vi "PointDetection-AnyPath.vi"() -> ()   [LabVIEW 2014]
doc: "This example shows how to use the Edge Tool in NI Vision. The Edge Tool finds edges (or sharp transitions in the pixels values) along a given line or ROI profile. The Edge Tool is a precursor function to many of the gauging and inspection tasks. For example, the location of the edges found along a line profile across an object can interpreted as the boundaries of the object whose dimensions have to be measured for a gauging application or the presence of a crack in the surface of an object for an inspection application."
uses:
  <vilib>/vision/NI_Vision_Development_Module.lvlib
panel:
  out "Number of Edges Detected":i32
  in  "Process":u16(ring)=2 items=["Get First Edge", "Get First + Last Edge", "Get All Edges", "Get Best Edge"]
  in  "Edge Options":T1={"Edge Polarity"=0, "Kernel Size"=3, "Width"=5, "Minimum Edge Strength"=10.0, "Interpolation Type"=1, "Data Processing Method"=0} {"Data Processing Method" items=["Average", "Median"]; "Interpolation Type" items=["Zero Order"=0, "Bilinear"=1, "Bilinear Fixed"=4]; "Minimum Edge Strength" min=0.0 max=255.0 format="%.2g"; "Width" min=1 step=2; "Kernel Size" min=3 step=2; "Edge Polarity" items=["All Edges", "Rising Edges", "Falling Edges"]}
  out "Gradient Information":dbl[](graph)
  out "Image":T2(plugin-control)
  out "Line Profile":cluster{"x0":sgl, "dx":sgl, "Pixels Line":sgl[]}(graph)
  in  "Stop":bool
  # "Overview: Demonstrates the edges detection along a Region of Interest (ROI).\nRequirements: Vision Development Software.\nInstructions: 1. Run the VI;  2. Change the Process or Edge Options to see the edges detected along the ROI."
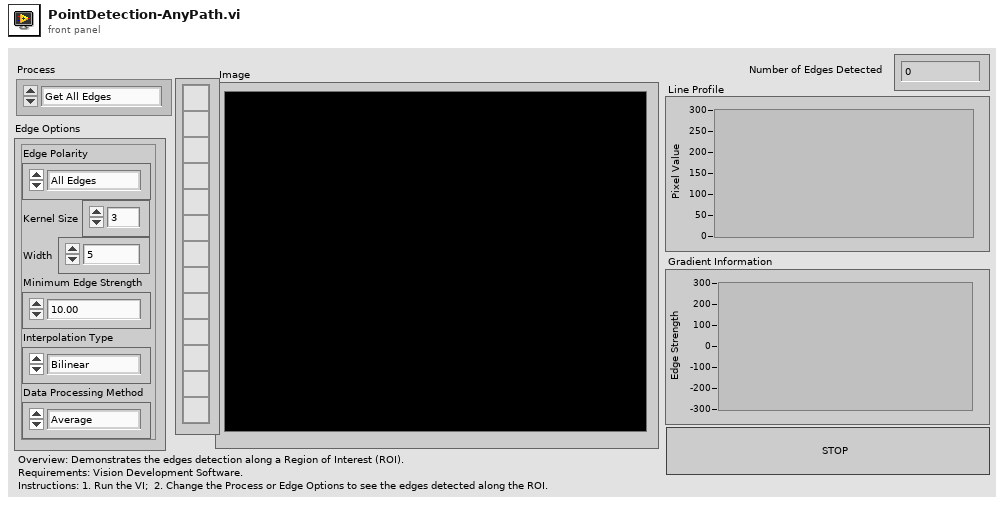
[diagram p1: front panel]
types:
  T1 = cluster{"Edge Polarity":u16, "Kernel Size":u32, "Width":u32, "Minimum Edge Strength":dbl, "Interpolation Type":u16, "Data Processing Method":u16}
  T2 = typedef "IMAQ Image.ctl" = refnum<image>
  T3 = typedef "IMAQ Line" = cluster{"Start X":i32, "Start Y":i32, "End X":i32, "End Y":i32}
  T4 = typedef "ROI Descriptor" = cluster{"Global Rectangle":i32[], "Contours":cluster{"ID":enum32{"External", "Internal"}, "Type":u32, "Coordinates":i32[]}[]}
  T5 = cluster{"Global Rectangle":i32[], "Contours":cluster{"Contour Type":u32, "ROI Type":u32, "Points":i32[]}[]}
  T6 = typedef "Edge New.ctl" = cluster{"Location (Pixel)":cluster{"X":sgl, "Y":sgl}, "Location (Real-World)":cluster{"X":sgl, "Y":sgl}, "Distance (Pixel)":dbl, "Distance (Real-World)":dbl, "Strength":dbl, "Noise":dbl, "Rising?":bool}
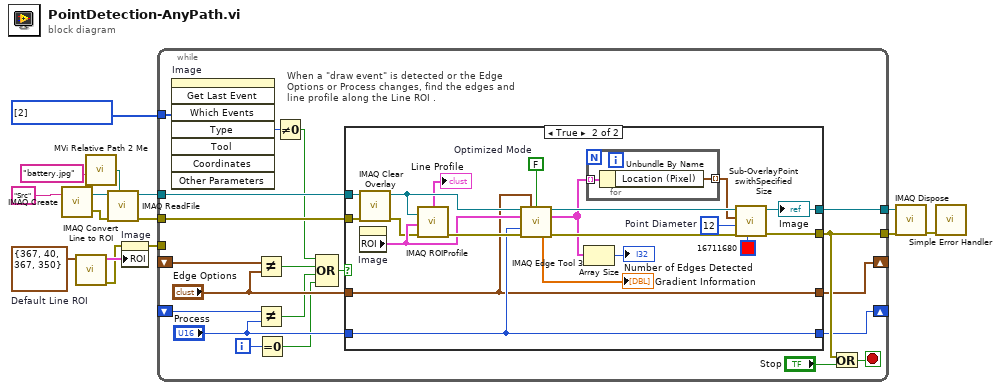
[diagram p0: block diagram]
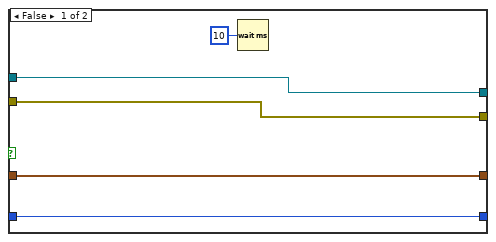
[diagram p2: hidden frame]
diagram:
  w3 = T3 {"Start X"=367, "Start Y"=40, "End X"=367, "End Y"=350}  # Default Line ROI
  w7 = i32[] [2] items=["No  event", "Click event", "Draw event", "Move event", "Size event", "Scroll event", "Activate event", "Close event", "Double click event"] ("Events list (all)")
  n1 = call "IMAQ Create"("Image Name"="Src") -> ("New Image"=w14:T2, "error out"=w13:errorcluster)  [unwired: 4 in]
  n2 = call "IMAQ Convert Line to ROI"("Line"=w3) -> ("error out"=w1:errorcluster, "ROI Descriptor"=w2:T4)  [unwired: 8 in]
  n3 = call "MVi Relative Path 2 Me.vi"("Relative Path"="battery.jpg" ("name or relative path")) -> ("Appended Dir"=w4:path)  [unwired: 5 in, 1 out]
  n4 = call "IMAQ ReadFile"("File Path"=w4, "error in (no error)"=w13, "Image"=w14) -> ("error out"=w8:errorcluster, "Image Out"=w9:T2)  [unwired: 4 in, 3 out]
  n5 = property on="Image" class="ImageControl"(error in=w1, "ROI"=w2) -> (error out=w6:errorcluster)  [unwired: 1 in, 1 out]
  n6 = while {
    tunnel: w9 -> [w34]
    tunnel: w8 -> [w35]
    tunnel: [w30] -> w12
    tunnel: [w31] -> w11
    tunnel: w7 -> [w29]
    shift-right: [w16] -> _
    shift-left: _ -> [w26]
    shift-right: [w17] -> _
    shift-left: _ -> [w24]
    tunnel: w6 -> [_]
    i -> [w27]
    stop <- w32 stop-if-true
    # "When a \"draw event\" is detected or the Edge Options or Process changes, find the edges and line profile along the Line ROI ."
    n7 = invoke on="Image" class="ImageControl" method="Get Last Event"("Which Events"=w29) -> ("Type"=w28:i32)  [unwired: 7 in, 7 out]
    n8 = Not Equal?(x=w26, y="Edge Options") -> (x != y?=w22:bool)
    n9 = Not Equal?(x=w24, y="Process") -> (x != y?=w21:bool)
    n10 = Equal To 0?(x=w27) -> (x = 0?=w20:bool)
    n11 = Not Equal To 0?(x=w28) -> (x != 0?=w19:bool)
    n12 = Compound Arithmetic op=OR(w19, w22, w21, w20) -> (w18:bool)
    n13 = case shown="True" w18 {
      tunnel: w35 -> [w39 w50]
      tunnel: w34 -> [w40 w49]
      tunnel: [w40 w52] -> w31
      tunnel: [w39 w56] -> w30
      tunnel: "Edge Options" -> [w37 w43]
      tunnel: "Process" -> [w36 w45]
      tunnel: [w36 w45] -> w17
      tunnel: [w37 w43] -> w16
      frame False {
        n14 = Wait (ms)(milliseconds to wait=u32 10) -> ()  [unwired: 1 out]
      }
      frame True {
        w41 = u32 12  # Point Diameter
        w46 = FALSE  # Optimized Mode
        n15 = call "IMAQ Clear Overlay"("error in (no error)"=w50, "Image"=w49) -> ("error out"=w47:errorcluster, "Image Out"=w48:T2)  [unwired: 8 in]
        n16 = property on="Image" class="ImageControl"() -> ("ROI"=w51:T5)  [unwired: 2 in, 2 out]
        n17 = call "IMAQ ROIProfile"("error in (no error)"=w47, "ROI Descriptor"=w51, "Image"=w48) -> ("error out"=w58:errorcluster, "ROI Graph"=→"Line Profile":cluster{"x0":sgl, "dx":sgl, "Pixels Line":sgl[]})  [unwired: 1 in, 3 out]
        n18 = call "IMAQ Edge Tool 3"("Image"=w48, "Edge Options"=w43, "Optimized Mode"=w46, "ROI Descriptor"=w51, "Process"=w45, "error in (no error)"=w58) -> ("Image (duplicate)"=w55:T2, "Edge Information"=w54:T6[], "Gradient Values"=→"Gradient Information":dbl[], "error out"=w57:errorcluster)  [unwired: 5 in, 1 out]
        n19 = Array Size(array=w54) -> (size(s)=→"Number of Edges Detected":i32)
        n20 = for {
          tunnel: w54 -> [w62] mode=indexing
          tunnel: [w61] -> w42 mode=indexing
          n21 = Unbundle By Name(w62) -> ("Location (Pixel)"=w61:cluster{"X":sgl, "Y":sgl})
        }
        n22 = call "Sub-OverlayPointswithSpecified Size.vi"("Color"=u32 16711680, "error in"=w57, "Point Diameter (5)"=w41, "Points"=w42, "Image In"=w55) -> ("error out"=w56:errorcluster, "Image Out"=w52:T2)  [unwired: 5 in]
        "Image" <- w52
      }
    }
    n23 = Or(x=w30, y="Stop") -> (x .or. y?=w32:bool)
  }
  n24 = call "IMAQ Dispose"("Image"=w11, "error in (no error)"=w12) -> ("error out"=w10:errorcluster)  [unwired: 4 in]
  n25 = call <vilib>:"Simple Error Handler.vi"("error in (no error)"=w10) -> ()  [unwired: 4 in, 5 out]
